vi "ExReadFileHeader.vi"(5 "error in (no error)":errorcluster) -> (4 "error out":errorcluster)   [LabVIEW 2010]
panel:
  in  "ROI Number":i16=1 min=1 max=1000 step=1
  in  "Point Pair":i16=1 min=1 max=1000 step=1
  out "Coefficient":dbl[](array[numeric]) format="%.10f"
  out "Laser Line (nm)":dbl format="%.3f"
  out "Display\nUnits":u32
  out "Polymonial\nUnits":u32
  out "Input Units":u32
  out "Adjust":dbl format="%.8f"
  out "Offset":dbl format="%.3f"
  out "Valid Calib":u32
  out "Calib Value":dbl format="%.5f"
  out "Pixel Number":dbl format="%.2f"
  out "Num Point Pairs":u32
  out "Max Point Pairs":u32
  out "Polynomial Order":u32
  out "Max Coeffs":u32
  out "On Detector\nAccumulations":u32
  out "Sequential\nPulse Delay\nEnd":dbl format="%.2f"
  out "Sequential\nPulse Delay\nStart":dbl format="%.2f"
  out "Sequential\nPulse Width\nEnd":dbl format="%.2f"
  out "Sequential\nPulse Width\nStart":dbl format="%.2f"
  out "Sequential\nInc Mode":u32
  out "Repetative\nPulse\nDelay":dbl format="%.2f"
  out "Repetative\nPulse\nWidth":dbl format="%.2f"
  out "Pulse Mode":u32
  out "Pulser Type":u32
  in  "Full File Name":path
  in  "FileType":u32=67371008
  out "Y Bin":u32
  out "Y End":u32
  out "Y Start":u32
  out "X Bin":u32
  out "X End":u32
  out "X Start":u32
  out "Max ROIs\nAllowed in\nFile Header":u32
  out "Current\nNumber\nof ROIs":u32
  out "Live\nAbsorbance\nApplied Flag":u32
  out "Flat Field\nApplied Flag":u32
  out "Live\nBackground\nSubtraction\nApplied Flag":u32
  out "Number of\nAccumulations":u32
  out "ADC Rate":u32
  out "External\nTrigger Flag":u32
  out "Triggered\nMode Flag":u32
  out "Shutter\nType":u32
  out "Camera\nType":u32
  out "Camera\nNumber":u32
  out "Intensifier\nGain":u32
  out "Intensifier\nGate Mode":u32
  out "Experiment\nTemperature":dbl format="%.2f"
  out "Exposure\n(seconds)":dbl format="%.2f"
  out "ADC\nOffset":u32
  out "Continuouse\nCleans Flag":u32
  out "Timing\nMode":u32
  out "Num Min\nBlocks":u32
  out "Min Block\nSize":u32
  out "Num Strips\nPer Clear":u32
  out "Number\nof Clears":u32
  out "Readout\nMode":u32
  out "Chip Y Size":u32
  out "Chip X Size":u32
  out "Logic Out":u32
  # "ExReadSpeFileHeader.vi\nThis VI will use read information stored in the file header and display it."
  # "File Types:\nSPE = 67371008\nTIF  = 67174400\nPMI = 67436544"
  # "Browse match pattern is set to *.spe.  Modify this if different file type is needed."
  # "CAMERA RELATED ITEMS"
  # "PULSER RELATED\n        ITEMS"
  # "CALIBRATION\nRELATED ITEMS"
  # "Regions Of\n  Interest"
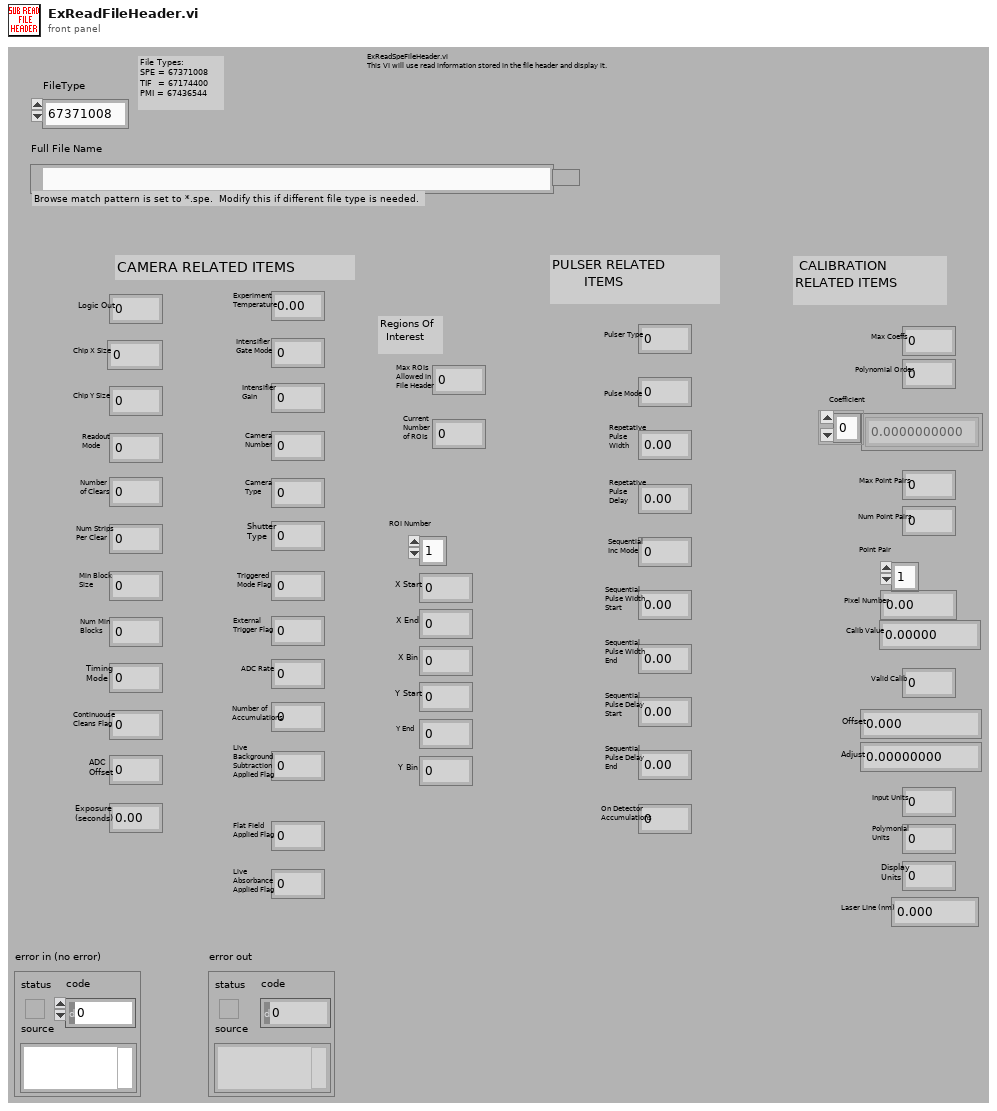
[diagram p1: front panel]
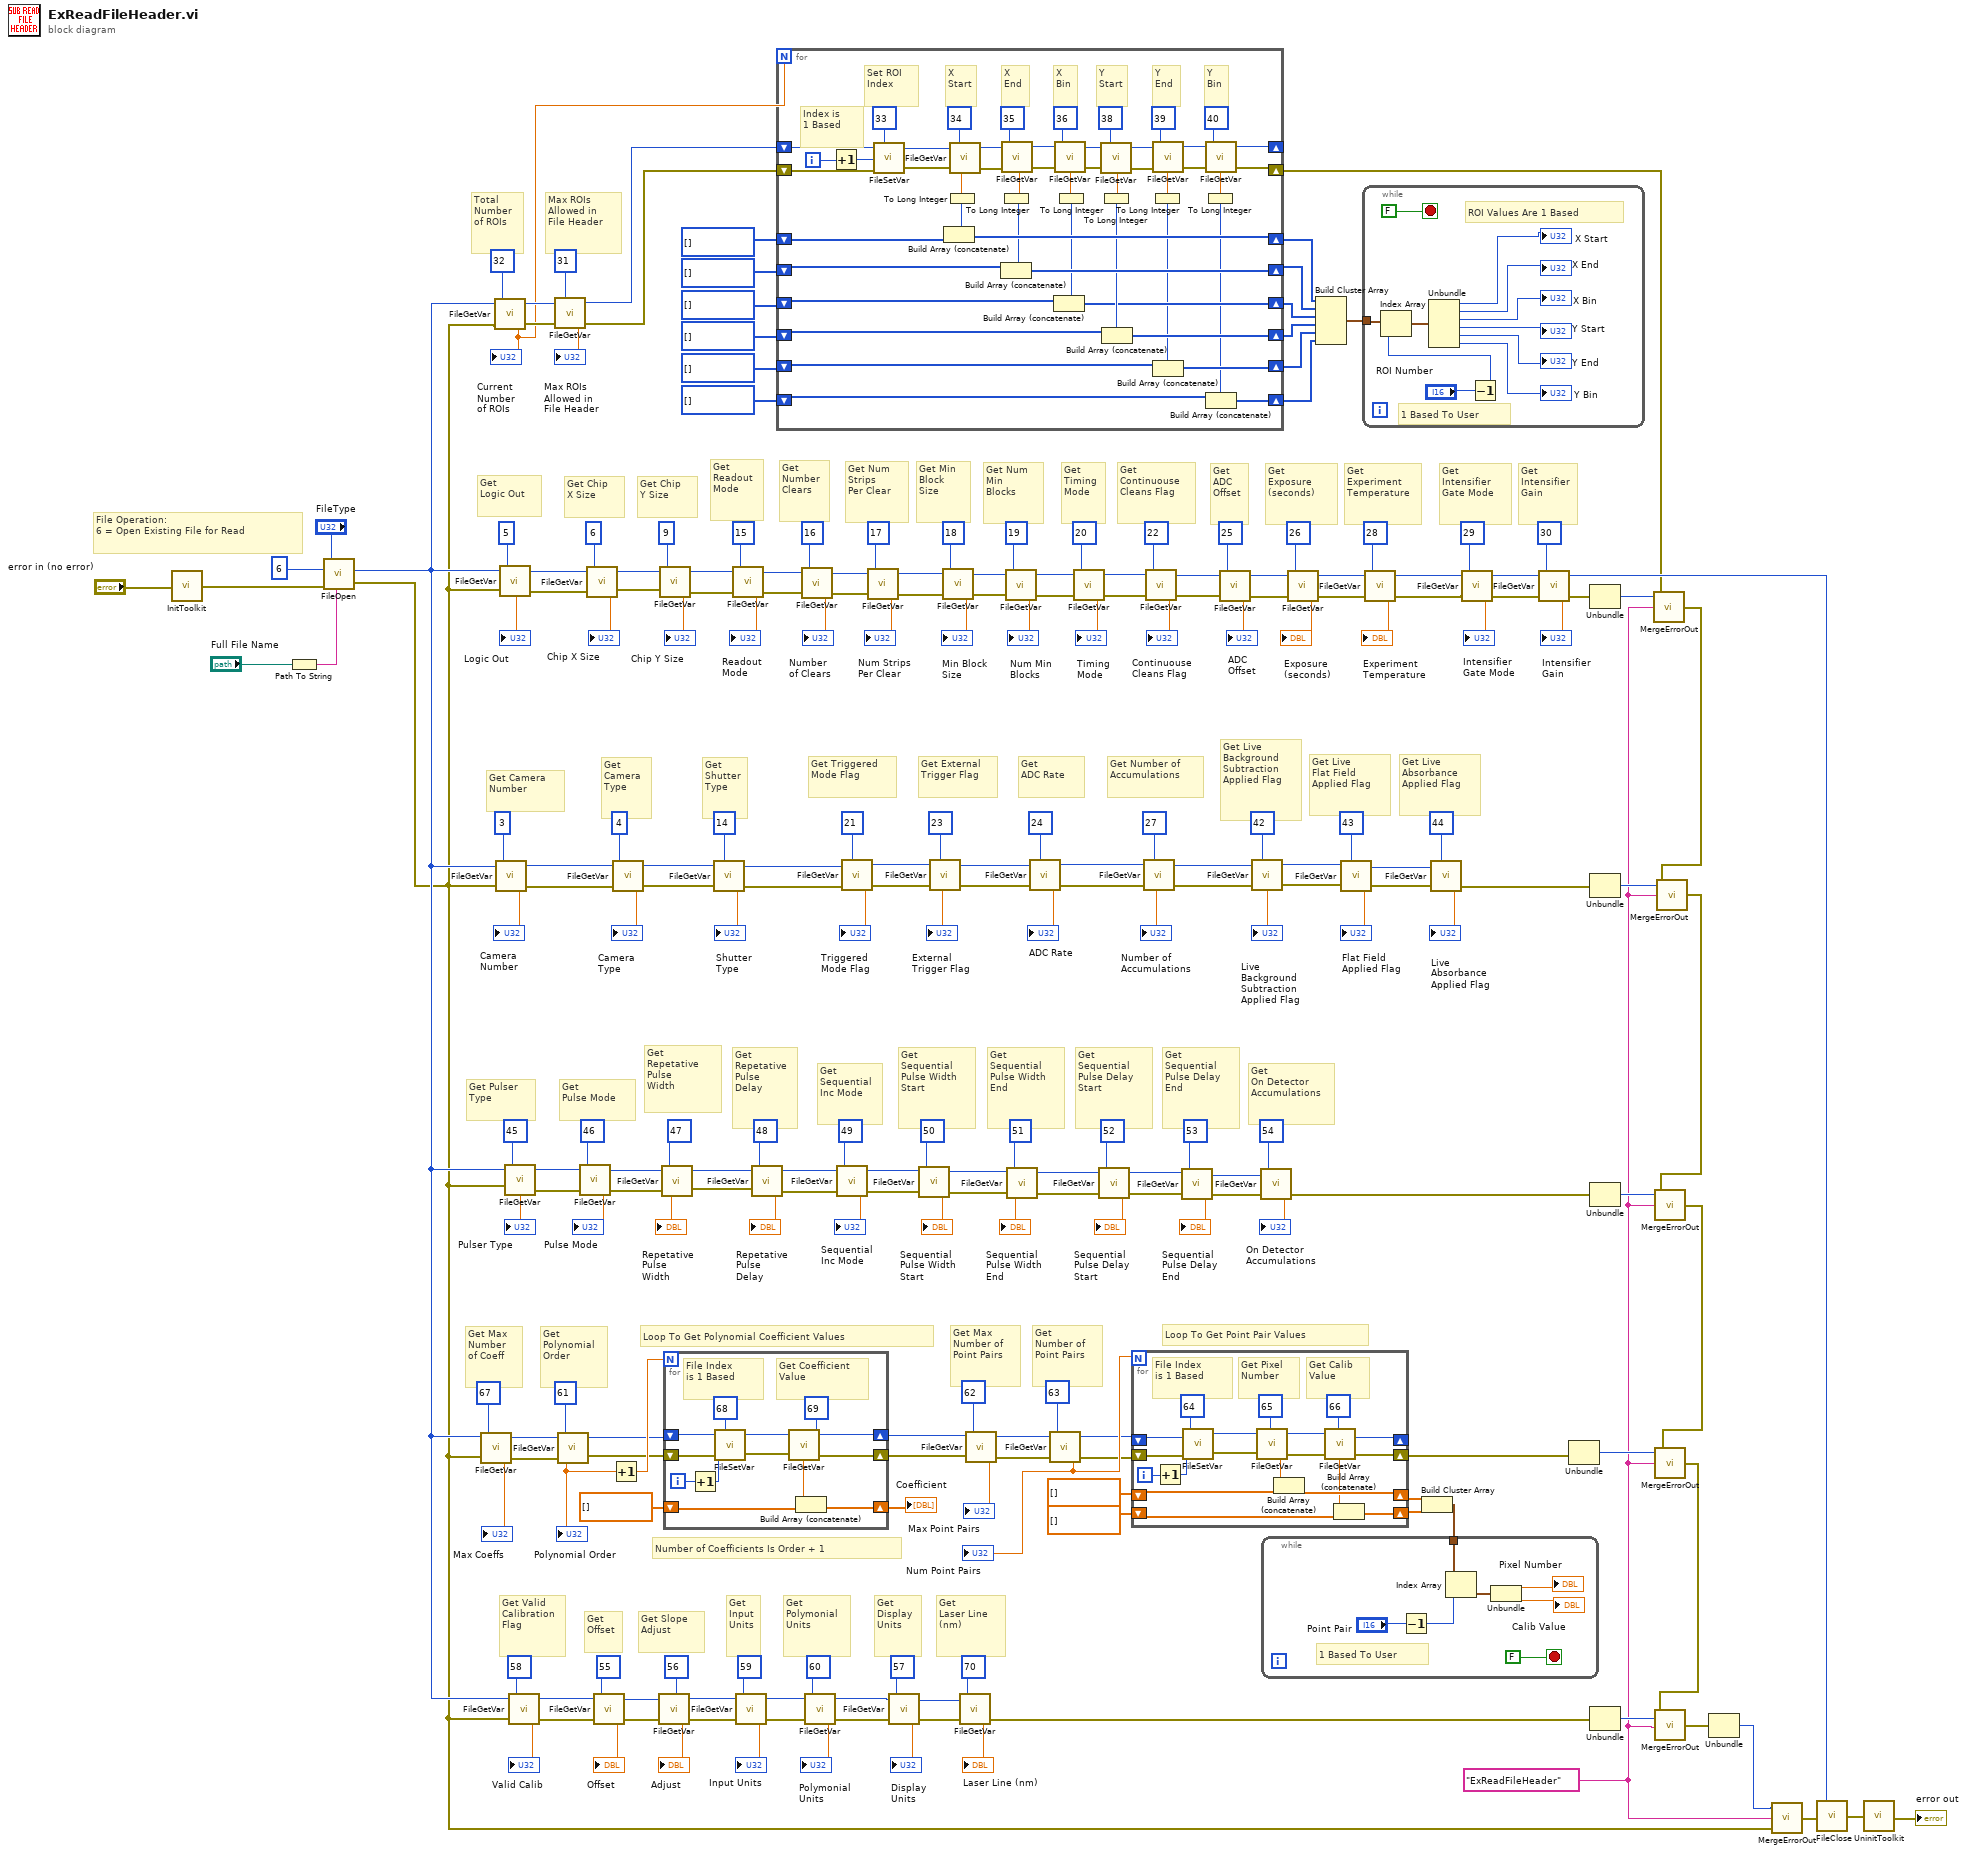
[diagram p0: block diagram]
diagram:
  w39 = "ExReadFileHeader"
  # "Loop To Get Point Pair Values"
  # "Get\nNumber of\nPoint Pairs"
  # "Get Max\nNumber of\nPoint Pairs"
  # "Loop To Get Polynomial Coefficient Values"
  # "Number of Coefficients Is Order + 1"
  # "Get\nPolynomial\nOrder"
  # "Get Max\nNumber\nof Coeff"
  # "Get\nPolymonial\nUnits"
  # "Get\nInput\nUnits"
  # "Get Slope\nAdjust"
  # "Get\nOffset"
  # "Get Valid\nCalibration\nFlag"
  # "Get\nLaser Line\n(nm)"
  # "Get\nDisplay\nUnits"
  # "Get Pulser\nType"
  # "Get \nOn Detector\nAccumulations"
  # "Get\nSequential\nPulse Delay\nEnd"
  # "Get\nSequential\nPulse Delay\nStart"
  # "Get\nSequential\nPulse Width\nEnd"
  # "Get\nSequential\nPulse Width\nStart"
  # "Get\nSequential\nInc Mode"
  # "Get\nRepetative\nPulse\nDelay"
  # "Get\nRepetative\nPulse\nWidth"
  # "Get\nPulse Mode"
  # "File Operation:\n6 = Open Existing File for Read"
  # "Get Live\nAbsorbance\nApplied Flag"
  # "Get Live\nFlat Field\nApplied Flag"
  # "Get Live\nBackground\nSubtraction\nApplied Flag"
  # "Get \nIntensifier\nGain"
  # "Get \nIntensifier\nGate Mode"
  # "Get Number of\nAccumulations"
  # "Get \nExperiment\nTemperature"
  # "Get \nExposure\n(seconds)"
  # "Get\nADC\nOffset"
  # "Get Camera\nNumber"
  # "Get\nADC Rate"
  # "Get \nContinuouse\nCleans Flag"
  # "Get \nTiming\nMode"
  # "Get External\nTrigger Flag"
  # "Get Num\nMin\nBlocks"
  # "Get Min\nBlock\nSize"
  # "Get Num\nStrips\nPer Clear"
  # "Get\nNumber\nClears"
  # "Get\nReadout\nMode"
  # "Get Triggered\nMode Flag"
  # "Get\nShutter\nType"
  # "Get\nCamera\nType"
  # "Get Chip\nY Size"
  # "Get Chip\nX Size"
  # "Get\nLogic Out"
  # "Max ROIs\nAllowed in\nFile Header"
  # "Total\nNumber\nof ROIs"
  n1 = call <userlib>:"InitToolkit.vi"("error in"="error in (no error)") -> ("error out"=w130:errorcluster)
  n2 = Path To String(path="Full File Name") -> (string=w129:string)
  n3 = call <userlib>:"FileOpen.vi"("error in"=w130, "File Operations"=u32 6 ("File Operation"), "FileName"=w129, "File Type"="FileType") -> ("error out"=w35:errorcluster, "File Handle"=w45:u32)
  n4 = call <userlib>:"FileGetVar.vi"("error in"=w35, "Parameter ID"=67, "File Handle"=w45) -> ("error out"=w65:errorcluster, "Value"=→"Max Coeffs":dbl, "File Handle"=w66:u32)
  n5 = call <userlib>:"FileGetVar.vi"("error in"=w35, "Parameter ID"=32, "File Handle"=w45) -> ("error out"=w234:errorcluster, "Value"=w14:dbl, "File Handle"=w235:u32)
  "Current\nNumber\nof ROIs" <- w14
  n6 = call <userlib>:"FileGetVar.vi"("error in"=w35, "Parameter ID"=3, "File Handle"=w45) -> ("error out"=w193:errorcluster, "Value"=→"Camera\nNumber":dbl, "File Handle"=w192:u32)
  n7 = call <userlib>:"FileGetVar.vi"("error in"=w35, "Parameter ID"=5, "File Handle"=w45) -> ("error out"=w227:errorcluster, "Value"=→"Logic Out":dbl, "File Handle"=w230:u32)
  n8 = call <userlib>:"FileGetVar.vi"("error in"=w35, "Parameter ID"=45, "File Handle"=w45) -> ("error out"=w94:errorcluster, "Value"=→"Pulser Type":dbl, "File Handle"=w93:u32)
  n9 = call <userlib>:"FileGetVar.vi"("error in"=w35, "Parameter ID"=58, "File Handle"=w45) -> ("error out"=w59:errorcluster, "Value"=→"Valid Calib":dbl, "File Handle"=w47:u32)
  n10 = call <userlib>:"FileGetVar.vi"("error in"=w234, "Parameter ID"=31, "File Handle"=w235) -> ("error out"=w16:errorcluster, "Value"=→"Max ROIs\nAllowed in\nFile Header":dbl, "File Handle"=w17:u32)
  n11 = call <userlib>:"FileGetVar.vi"("error in"=w65, "Parameter ID"=61, "File Handle"=w66) -> ("error out"=w30:errorcluster, "Value"=w60:dbl, "File Handle"=w31:u32)
  "Polynomial Order" <- w60
  n12 = call <userlib>:"FileGetVar.vi"("error in"=w94, "Parameter ID"=46, "File Handle"=w93) -> ("error out"=w116:errorcluster, "Value"=→"Pulse Mode":dbl, "File Handle"=w119:u32)
  n13 = call <userlib>:"FileGetVar.vi"("error in"=w227, "Parameter ID"=6, "File Handle"=w230) -> ("error out"=w228:errorcluster, "Value"=→"Chip X Size":dbl, "File Handle"=w229:u32)
  n14 = call <userlib>:"FileGetVar.vi"("error in"=w59, "Parameter ID"=55, "File Handle"=w47) -> ("error out"=w73:errorcluster, "Value"=→"Offset":dbl, "File Handle"=w74:u32)
  n15 = Increment(x=w60) -> (x+1=w34:dbl)
  n16 = call <userlib>:"FileGetVar.vi"("error in"=w193, "Parameter ID"=4, "File Handle"=w192) -> ("error out"=w217:errorcluster, "Value"=→"Camera\nType":dbl, "File Handle"=w220:u32)
  n17 = call <userlib>:"FileGetVar.vi"("error in"=w73, "Parameter ID"=56, "File Handle"=w74) -> ("error out"=w58:errorcluster, "Value"=→"Adjust":dbl, "File Handle"=w46:u32)
  n18 = call <userlib>:"FileGetVar.vi"("error in"=w228, "Parameter ID"=9, "File Handle"=w229) -> ("error out"=w221:errorcluster, "Value"=→"Chip Y Size":dbl, "File Handle"=w222:u32)
  n19 = call <userlib>:"FileGetVar.vi"("error in"=w116, "Parameter ID"=47, "File Handle"=w119) -> ("error out"=w117:errorcluster, "Value"=→"Repetative\nPulse\nWidth":dbl, "File Handle"=w118:u32)
  n20 = for {
    N: w34 -> [_]
    shift-right: [w244] -> w32
    shift-left: w31 -> [w243]
    shift-right: [w241] -> w29
    shift-left: w30 -> [w242]
    shift-right: [w240] -> w27
    shift-left: dbl[] [] -> [w239]
    i -> [w245]
    # "Get Coefficient\nValue"
    # "File Index\nis 1 Based"
    n21 = Increment(x=w245) -> (x+1=w246:i32)
    n22 = call <userlib>:"FileSetVar.vi"("error in"=w242, "Value"=w246, "Parameter ID"=68, "File Handle"=w243) -> ("error out"=w249:errorcluster, "File Handle"=w248:u32)
    n23 = call <userlib>:"FileGetVar.vi"("error in"=w249, "Parameter ID"=69, "File Handle"=w248) -> ("error out"=w241:errorcluster, "Value"=w238:dbl, "File Handle"=w244:u32)
    n24 = Build Array (concatenate)(w239, w238) -> (w240:dbl[])
  }
  "Coefficient" <- w27
  n25 = call <userlib>:"FileGetVar.vi"("error in"=w217, "Parameter ID"=14, "File Handle"=w220) -> ("error out"=w218:errorcluster, "Value"=→"Shutter\nType":dbl, "File Handle"=w219:u32)
  n26 = call <userlib>:"FileGetVar.vi"("error in"=w221, "Parameter ID"=15, "File Handle"=w222) -> ("error out"=w208:errorcluster, "Value"=→"Readout\nMode":dbl, "File Handle"=w212:u32)
  n27 = call <userlib>:"FileGetVar.vi"("error in"=w58, "Parameter ID"=59, "File Handle"=w46) -> ("error out"=w57:errorcluster, "Value"=→"Input Units":dbl, "File Handle"=w69:u32)
  n28 = call <userlib>:"FileGetVar.vi"("error in"=w117, "Parameter ID"=48, "File Handle"=w118) -> ("error out"=w113:errorcluster, "Value"=→"Repetative\nPulse\nDelay":dbl, "File Handle"=w114:u32)
  n29 = for {
    N: w14 -> [_]
    shift-right: [w279] -> _
    shift-left: w17 -> [w280]
    shift-right: [w277] -> w15
    shift-left: w16 -> [w278]
    shift-right: [w273] -> w7
    shift-left: i32[] [] -> [w274]
    shift-right: [w267] -> w6
    shift-left: i32[] [] -> [w270]
    shift-right: [w261] -> w5
    shift-left: i32[] [] -> [w265]
    shift-right: [w259] -> w4
    shift-left: i32[] [] -> [w260]
    shift-right: [w255] -> w3
    shift-left: i32[] [] -> [w257]
    shift-right: [w251] -> w2
    shift-left: i32[] [] -> [w253]
    i -> [w276]
    # "Y\nBin"
    # "Y\nEnd"
    # "Y\nStart"
    # "X\nBin"
    # "X\nEnd"
    # "X\nStart"
    # "Index is\n1 Based"
    # "Set ROI\nIndex"
    n30 = Increment(x=w276) -> (x+1=w275:i32)
    n31 = call <userlib>:"FileSetVar.vi"("error in"=w278, "Value"=w275, "Parameter ID"=33, "File Handle"=w280) -> ("error out"=w292:errorcluster, "File Handle"=w295:u32)
    n32 = call <userlib>:"FileGetVar.vi"("error in"=w292, "Parameter ID"=34, "File Handle"=w295) -> ("error out"=w291:errorcluster, "Value"=w272:dbl, "File Handle"=w294:u32)
    n33 = To Long Integer(number=w272) -> (32bit integer=w271:i32)
    n34 = Build Array (concatenate)(w274, w271) -> (w273:i32[])
    n35 = call <userlib>:"FileGetVar.vi"("error in"=w291, "Parameter ID"=35, "File Handle"=w294) -> ("error out"=w290:errorcluster, "Value"=w269:dbl, "File Handle"=w293:u32)
    n36 = To Long Integer(number=w269) -> (32bit integer=w268:i32)
    n37 = Build Array (concatenate)(w270, w268) -> (w267:i32[])
    n38 = call <userlib>:"FileGetVar.vi"("error in"=w290, "Parameter ID"=36, "File Handle"=w293) -> ("error out"=w281:errorcluster, "Value"=w264:dbl, "File Handle"=w282:u32)
    n39 = To Long Integer(number=w264) -> (32bit integer=w266:i32)
    n40 = Build Array (concatenate)(w265, w266) -> (w261:i32[])
    n41 = call <userlib>:"FileGetVar.vi"("error in"=w281, "Parameter ID"=38, "File Handle"=w282) -> ("error out"=w284:errorcluster, "Value"=w262:dbl, "File Handle"=w286:u32)
    n42 = To Long Integer(number=w262) -> (32bit integer=w263:i32)
    n43 = Build Array (concatenate)(w260, w263) -> (w259:i32[])
    n44 = call <userlib>:"FileGetVar.vi"("error in"=w284, "Parameter ID"=39, "File Handle"=w286) -> ("error out"=w283:errorcluster, "Value"=w256:dbl, "File Handle"=w285:u32)
    n45 = To Long Integer(number=w256) -> (32bit integer=w258:i32)
    n46 = Build Array (concatenate)(w257, w258) -> (w255:i32[])
    n47 = call <userlib>:"FileGetVar.vi"("error in"=w283, "Parameter ID"=40, "File Handle"=w285) -> ("error out"=w277:errorcluster, "Value"=w252:dbl, "File Handle"=w279:u32)
    n48 = To Long Integer(number=w252) -> (32bit integer=w254:i32)
    n49 = Build Array (concatenate)(w253, w254) -> (w251:i32[])
  }
  n50 = call <userlib>:"FileGetVar.vi"("error in"=w208, "Parameter ID"=16, "File Handle"=w212) -> ("error out"=w207:errorcluster, "Value"=→"Number\nof Clears":dbl, "File Handle"=w211:u32)
  n51 = call <userlib>:"FileGetVar.vi"("error in"=w57, "Parameter ID"=60, "File Handle"=w69) -> ("error out"=w36:errorcluster, "Value"=→"Polymonial\nUnits":dbl, "File Handle"=w37:u32)
  n52 = call <userlib>:"FileGetVar.vi"("error in"=w113, "Parameter ID"=49, "File Handle"=w114) -> ("error out"=w104:errorcluster, "Value"=→"Sequential\nInc Mode":dbl, "File Handle"=w108:u32)
  n53 = call <userlib>:"FileGetVar.vi"("error in"=w218, "Parameter ID"=21, "File Handle"=w219) -> ("error out"=w196:errorcluster, "Value"=→"Triggered\nMode Flag":dbl, "File Handle"=w197:u32)
  n54 = call <userlib>:"FileGetVar.vi"("error in"=w207, "Parameter ID"=17, "File Handle"=w211) -> ("error out"=w206:errorcluster, "Value"=→"Num Strips\nPer Clear":dbl, "File Handle"=w210:u32)
  n55 = call <userlib>:"FileGetVar.vi"("error in"=w36, "Parameter ID"=57, "File Handle"=w37) -> ("error out"=w77:errorcluster, "Value"=→"Display\nUnits":dbl, "File Handle"=w76:u32)
  n56 = call <userlib>:"FileGetVar.vi"("error in"=w104, "Parameter ID"=50, "File Handle"=w108) -> ("error out"=w103:errorcluster, "Value"=→"Sequential\nPulse Width\nStart":dbl, "File Handle"=w107:u32)
  n57 = call <userlib>:"FileGetVar.vi"("error in"=w196, "Parameter ID"=23, "File Handle"=w197) -> ("error out"=w190:errorcluster, "Value"=→"External\nTrigger Flag":dbl, "File Handle"=w191:u32)
  n58 = call <userlib>:"FileGetVar.vi"("error in"=w206, "Parameter ID"=18, "File Handle"=w210) -> ("error out"=w205:errorcluster, "Value"=→"Min Block\nSize":dbl, "File Handle"=w209:u32)
  n59 = call <userlib>:"FileGetVar.vi"("error in"=w77, "Parameter ID"=70, "File Handle"=w76) -> ("error out"=w42:errorcluster, "Value"=→"Laser Line (nm)":dbl)  [unwired: 1 out]
  n60 = call <userlib>:"FileGetVar.vi"("error in"=w29, "Parameter ID"=62, "File Handle"=w32) -> ("error out"=w61:errorcluster, "Value"=→"Max Point Pairs":dbl, "File Handle"=w62:u32)
  n61 = call <userlib>:"FileGetVar.vi"("error in"=w205, "Parameter ID"=19, "File Handle"=w209) -> ("error out"=w199:errorcluster, "Value"=→"Num Min\nBlocks":dbl, "File Handle"=w201:u32)
  n62 = call <userlib>:"FileGetVar.vi"("error in"=w103, "Parameter ID"=51, "File Handle"=w107) -> ("error out"=w102:errorcluster, "Value"=→"Sequential\nPulse Width\nEnd":dbl, "File Handle"=w106:u32)
  n63 = call <userlib>:"FileGetVar.vi"("error in"=w190, "Parameter ID"=24, "File Handle"=w191) -> ("error out"=w178:errorcluster, "Value"=→"ADC Rate":dbl, "File Handle"=w179:u32)
  n64 = call <userlib>:"FileGetVar.vi"("error in"=w61, "Parameter ID"=63, "File Handle"=w62) -> ("error out"=w22:errorcluster, "Value"=w33:dbl, "File Handle"=w20:u32)
  "Num Point Pairs" <- w33
  n65 = call <userlib>:"FileGetVar.vi"("error in"=w199, "Parameter ID"=20, "File Handle"=w201) -> ("error out"=w198:errorcluster, "Value"=→"Timing\nMode":dbl, "File Handle"=w200:u32)
  n66 = call <userlib>:"FileGetVar.vi"("error in"=w102, "Parameter ID"=52, "File Handle"=w106) -> ("error out"=w101:errorcluster, "Value"=→"Sequential\nPulse Delay\nStart":dbl, "File Handle"=w105:u32)
  n67 = for {
    N: w33 -> [_]
    shift-right: [w307] -> w24
    shift-left: dbl[] [] -> [w309]
    shift-right: [w304] -> w23
    shift-left: dbl[] [] -> [w306]
    shift-right: [w302] -> w21
    shift-left: w22 -> [w303]
    shift-right: [w300] -> _
    shift-left: w20 -> [w301]
    i -> [w310]
    # "Get Calib\nValue"
    # "Get Pixel\nNumber"
    # "File Index\nis 1 Based"
    n68 = Increment(x=w310) -> (x+1=w318:i32)
    n69 = call <userlib>:"FileSetVar.vi"("error in"=w303, "Value"=w318, "Parameter ID"=64, "File Handle"=w301) -> ("error out"=w316:errorcluster, "File Handle"=w315:u32)
    n70 = call <userlib>:"FileGetVar.vi"("error in"=w316, "Parameter ID"=65, "File Handle"=w315) -> ("error out"=w311:errorcluster, "Value"=w308:dbl, "File Handle"=w312:u32)
    n71 = Build Array (concatenate)(w309, w308) -> (w307:dbl[])
    n72 = call <userlib>:"FileGetVar.vi"("error in"=w311, "Parameter ID"=66, "File Handle"=w312) -> ("error out"=w302:errorcluster, "Value"=w305:dbl, "File Handle"=w300:u32)
    n73 = Build Array (concatenate)(w306, w305) -> (w304:dbl[])
  }
  n74 = call <userlib>:"FileGetVar.vi"("error in"=w178, "Parameter ID"=27, "File Handle"=w179) -> ("error out"=w165:errorcluster, "Value"=→"Number of\nAccumulations":dbl, "File Handle"=w168:u32)
  n75 = call <userlib>:"FileGetVar.vi"("error in"=w198, "Parameter ID"=22, "File Handle"=w200) -> ("error out"=w181:errorcluster, "Value"=→"Continuouse\nCleans Flag":dbl, "File Handle"=w182:u32)
  n76 = call <userlib>:"FileGetVar.vi"("error in"=w101, "Parameter ID"=53, "File Handle"=w105) -> ("error out"=w98:errorcluster, "Value"=→"Sequential\nPulse Delay\nEnd":dbl, "File Handle"=w99:u32)
  n77 = call <userlib>:"FileGetVar.vi"("error in"=w181, "Parameter ID"=25, "File Handle"=w182) -> ("error out"=w184:errorcluster, "Value"=→"ADC\nOffset":dbl, "File Handle"=w186:u32)
  n78 = call <userlib>:"FileGetVar.vi"("error in"=w165, "Parameter ID"=42, "File Handle"=w168) -> ("error out"=w164:errorcluster, "Value"=→"Live\nBackground\nSubtraction\nApplied Flag":dbl, "File Handle"=w167:u32)
  n79 = call <userlib>:"FileGetVar.vi"("error in"=w98, "Parameter ID"=54, "File Handle"=w99) -> ("error out"=w95:errorcluster, "Value"=→"On Detector\nAccumulations":dbl)  [unwired: 1 out]
  n80 = call <userlib>:"FileGetVar.vi"("error in"=w184, "Parameter ID"=26, "File Handle"=w186) -> ("error out"=w183:errorcluster, "Value"=→"Exposure\n(seconds)":dbl, "File Handle"=w185:u32)
  n81 = Build Cluster Array(w7, w6, w5, w4, w3, w2) -> (w1:cluster{i32, i32, i32, i32, i32, i32}[])
  n82 = call <userlib>:"FileGetVar.vi"("error in"=w164, "Parameter ID"=43, "File Handle"=w167) -> ("error out"=w163:errorcluster, "Value"=→"Flat Field\nApplied Flag":dbl, "File Handle"=w166:u32)
  n83 = while {
    tunnel: w1 -> [w325]
    stop <- FALSE stop-if-true
    # "ROI Values Are 1 Based"
    # "1 Based To User"
    n84 = Decrement(x="ROI Number") -> (x-1=w327:i16)
    n85 = Index Array(array=w325, index=w327) -> (element=w329:cluster{i32, i32, i32, i32, i32, i32})
    n86 = Unbundle(w329) -> (→"X Start":i32, →"X End":i32, →"X Bin":i32, →"Y Start":i32, →"Y End":i32, →"Y Bin":i32)
  }
  n87 = call <userlib>:"FileGetVar.vi"("error in"=w183, "Parameter ID"=28, "File Handle"=w185) -> ("error out"=w172:errorcluster, "Value"=→"Experiment\nTemperature":dbl, "File Handle"=w173:u32)
  n88 = Build Cluster Array(w24, w23) -> (w19:cluster{dbl, dbl}[])
  n89 = while {
    tunnel: w19 -> [w331]
    stop <- FALSE stop-if-true
    # "1 Based To User"
    n90 = Decrement(x="Point Pair") -> (x-1=w333:i16)
    n91 = Index Array(array=w331, index=w333) -> (element=w336:cluster{dbl, dbl})
    n92 = Unbundle(w336) -> (→"Pixel Number":dbl, →"Calib Value":dbl)
  }
  n93 = call <userlib>:"FileGetVar.vi"("error in"=w163, "Parameter ID"=44, "File Handle"=w166) -> ("error out"=w134:errorcluster, "Value"=→"Live\nAbsorbance\nApplied Flag":dbl)  [unwired: 1 out]
  n94 = call <userlib>:"FileGetVar.vi"("error in"=w172, "Parameter ID"=29, "File Handle"=w173) -> ("error out"=w174:errorcluster, "Value"=→"Intensifier\nGate Mode":dbl, "File Handle"=w175:u32)
  n95 = call <userlib>:"FileGetVar.vi"("error in"=w174, "Parameter ID"=30, "File Handle"=w175) -> ("error out"=w162:errorcluster, "Value"=→"Intensifier\nGain":dbl, "File Handle"=w123:u32)
  n96 = Unbundle(w21) -> ("code"=w44:i32)  [unwired: 2 out]
  n97 = Unbundle(w162) -> ("code"=w161:i32)  [unwired: 2 out]
  n98 = Unbundle(w134) -> ("code"=w133:i32)  [unwired: 2 out]
  n99 = Unbundle(w95) -> ("code"=w96:i32)  [unwired: 2 out]
  n100 = Unbundle(w42) -> ("code"=w41:i32)  [unwired: 2 out]
  n101 = call <userlib>:"MergeErrorOut.vi"("error in"=w15, "Fucntion Name"=w39, "ErrorCode"=w161) -> ("error out"=w132:errorcluster)
  n102 = call <userlib>:"MergeErrorOut.vi"("error in"=w132, "Fucntion Name"=w39, "ErrorCode"=w133) -> ("error out"=w82:errorcluster)
  n103 = call <userlib>:"MergeErrorOut.vi"("error in"=w82, "Fucntion Name"=w39, "ErrorCode"=w96) -> ("error out"=w43:errorcluster)
  n104 = call <userlib>:"MergeErrorOut.vi"("error in"=w43, "Fucntion Name"=w39, "ErrorCode"=w44) -> ("error out"=w40:errorcluster)
  n105 = call <userlib>:"MergeErrorOut.vi"("error in"=w40, "Fucntion Name"=w39, "ErrorCode"=w41) -> ("error out"=w38:errorcluster)
  n106 = Unbundle(w38) -> ("code"=w81:i32)  [unwired: 2 out]
  n107 = call <userlib>:"MergeErrorOut.vi"("error in"=w35, "Fucntion Name"=w39, "ErrorCode"=w81) -> ("error out"=w125:errorcluster)
  n108 = call <userlib>:"FileClose.vi"("error in"=w125, "File Handle"=w123) -> ("error out"=w18:errorcluster)
  n109 = call <userlib>:"UninitToolkit.vi"("error in"=w18) -> ("error out"=→"error out":errorcluster)
